vi "get_param_from_repo.vi"(8 "error in (no error)":errorcluster, 9 "param_name":string, 10 "repo_type":string, 11 "node in":refnum<k20>) -> (0 "error out":errorcluster, 2 "parameter":string, 3 "node out":refnum<k20>)   [LabVIEW 2010, in "XML_repo_library.lvlib"]
uses:
  XML_repo_library.lvlib
  <vilib>/xml/Close Reference(Node).vi
  <vilib>/xml/NI_XML.lvlib
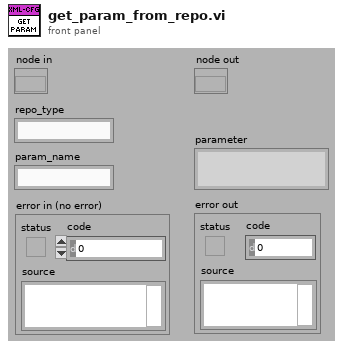
[diagram p1: front panel]
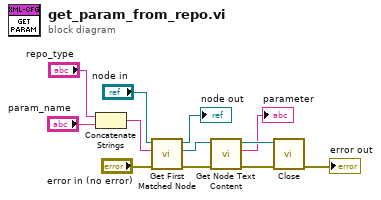
[diagram p0: block diagram]
diagram:
  n1 = Concatenate Strings("repo_type", "param_name") -> (w8:string)
  n2 = call <vilib>:"Get First Matched Node.vi"("error in (no error)"="error in (no error)", "XPath expression"=w8, "node in"="node in") -> ("error out"=w9:errorcluster, "node result"=w12:refnum<k20>, "node out"=→"node out":refnum<k20>)  [unwired: 6 in]
  n3 = call <vilib>:"Get Node Text Content.vi"("error in (no error)"=w9, "node in"=w12) -> ("error out"=w10:errorcluster, "node text"=→"parameter":string, "node out"=w11:refnum<k20>)  [unwired: 7 in]
  n4 = call-poly <vilib>:"Close.vi"("error in (no error)"=w10, "node"=w11) -> ("error out"=→"error out":errorcluster)  [unwired: 7 in]
